vi "Autodetect Board (SubVI).vi"(8 "error in (no error)":errorcluster, 11 "instr name":string="Arduino" caption="Board Name") -> (0 "error out":errorcluster, 2 "status":bool, 3 "VISA Refnum out":refnum<visa-resource-name>)   [LabVIEW 2015]
uses:
  <vilib>/Instr/_visa.llb/VISA Find Search Mode.ctl
  <vilib>/regexp/Match Regular Expression.xnode
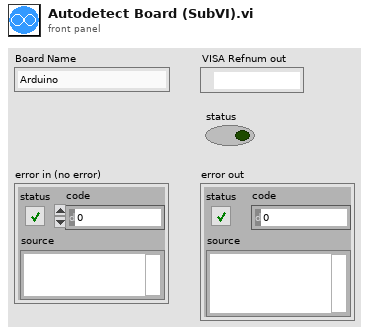
[diagram p1: front panel]
types:
  T1 = typedef "VISA Find Search Mode.ctl" = u32
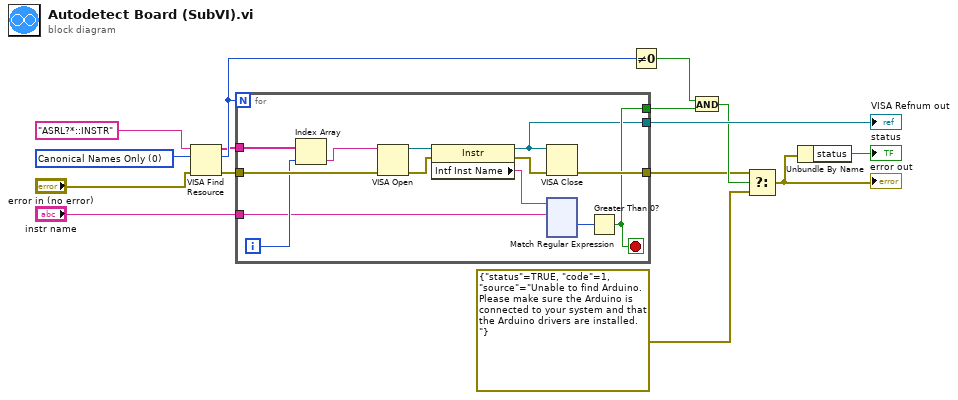
[diagram p0: block diagram]
diagram:
  w4 = T1 0 items=["Canonical Names Only"=0, "Aliases Only"=2, "Include Matching Aliases"=3, "Include All Aliases"=4] ("Search Mode")
  n1 = VISA Find Resource(8:"error in (no error)", 10:w4, 11:"ASRL?*::INSTR" ("expression (\"?*\")")) -> (0:w2:errorcluster, 2:w11:u32, 3:w3:string[])
  n2 = for {
    N: w11 -> [_]
    tunnel: w2 -> [w28]
    tunnel: w3 -> [w24]
    tunnel: [w21] -> w5
    tunnel: "instr name" -> [w19]
    tunnel: [w17] -> w8
    tunnel: [w16] -> w13
    i -> [w23]
    stop <- w17 stop-if-true
    n3 = Index Array(array=w24, index=w23) -> (element=w22:string)
    n4 = VISA Open(error in (no error)=w28, VISA resource name=w22) -> (VISA resource name=w25:refnum<visa-resource-name>, error out=w27:errorcluster)  [unwired: 3 in]
    n5 = property class="Instr"(reference=w25, error in=w27) -> (reference out=w16:refnum<visa-resource-name>, error out=w26:errorcluster, "Intf Inst Name"=w20:string)
    n6 = VISA Close(VISA resource name=w16, error in (no error)=w26) -> (error out=w21:errorcluster)
    n7 = xnode "Match Regular Expression"("input string"=w20, "regular expression"=w19) -> ("offset past match"=w18:i32)  [unwired: 4 in, 4 out]
    n8 = Greater Than 0?(x=w18) -> (x > 0?=w17:bool)
  }
  "VISA Refnum out" <- w13
  n9 = Not Equal To 0?(x=w11) -> (x != 0?=w6:bool)
  n10 = And(x=w6, y=w8) -> (x .and. y?=w9:bool)
  n11 = Select(t=w5, s=w9, f=errorcluster {"status"=TRUE, "code"=1, "source"="Unable to find Arduino.  Please make sure the Arduino is connected to your system and that the Arduino drivers are installed."}) -> (s? t:f=w14:errorcluster)
  "error out" <- w14
  n12 = Unbundle By Name(w14) -> ("status"=→"status":bool)
